vi "PID_control.vi"(10 "PID Gains":T1={"Proportional Gain (Kc)"=0.8, "Integral Gain"=25.0, "Derivative Gain"=0.004}, 11 "Gx, Gy, wz":dbl[](array[numeric])) -> (3 "PID %Power":T2)   [LabVIEW 2019]
panel:
  out "error out 2":errorcluster
  out "error out":errorcluster
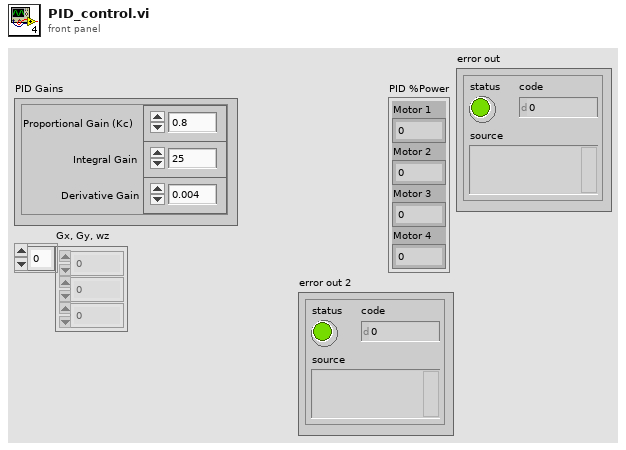
[diagram p1: front panel]
types:
  T1 = cluster{"Proportional Gain (Kc)":dbl, "Integral Gain":dbl, "Derivative Gain":dbl}
  T2 = cluster{"Motor 1":dbl, "Motor 2":dbl, "Motor 3":dbl, "Motor 4":dbl}
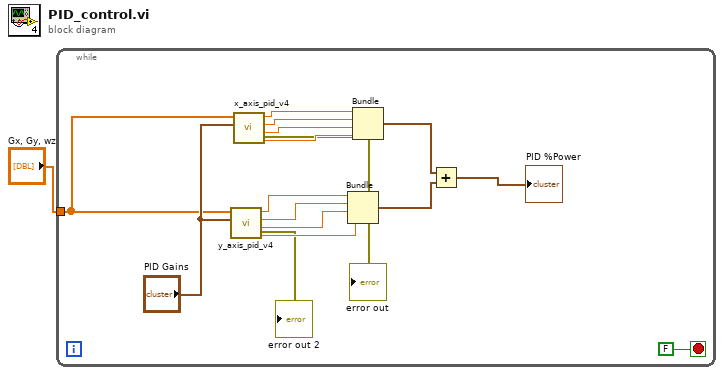
[diagram p0: block diagram]
diagram:
  n1 = while {
    tunnel: "Gx, Gy, wz" -> [w5]
    stop <- FALSE stop-if-true
    n2 = call "y_axis_pid_v4.vi"("PID Gains"="PID Gains", "Gx, Gy, wz"=w5) -> ("Motor 4"=w10:dbl, "Motor 3"=w11:dbl, "Motor 2"=w12:dbl, "Motor 1"=w13:dbl, "error out"=→"error out 2":errorcluster)  [unwired: 5 in]
    n3 = call "x_axis_pid_v4.vi"("PID Gains"="PID Gains", "Gx, Gy, wz"=w5) -> ("Motor 4"=w14:dbl, "Motor 3"=w15:dbl, "Motor 2"=w16:dbl, "Motor 1"=w17:dbl, "error out"=→"error out":errorcluster)  [unwired: 5 in]
    n4 = Bundle("Motor 1"=w13, "Motor 2"=w12, "Motor 3"=w11, "Motor 4"=w10) -> (w8:T2)  [unwired: 1 in]
    n5 = Bundle("Motor 1"=w17, "Motor 2"=w16, "Motor 3"=w15, "Motor 4"=w14) -> (w9:T2)  [unwired: 1 in]
    n6 = Add(x=w9, y=w8) -> (x+y=→"PID %Power":T2)
  }
